vi "Ej_13_DAQ_Escritura_Digital.vi"() -> ()   [LabVIEW 2021]
panel:
  in  "lower limit":dbl
  in  "upper limit":dbl
  out "Temperatura":dbl
  in  "stop":bool
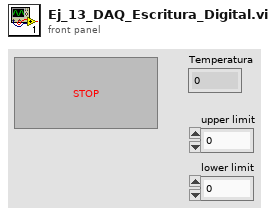
[diagram p1: front panel]
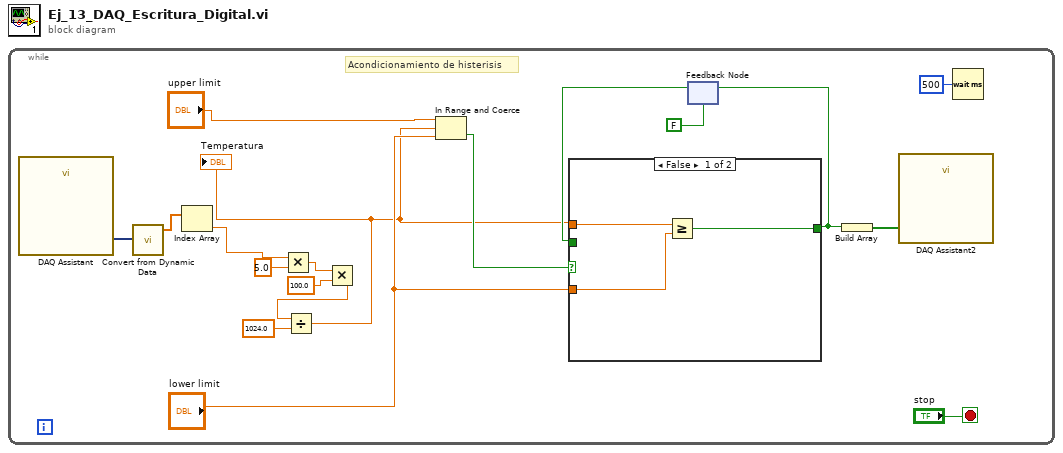
[diagram p0: block diagram]
diagram:
  n1 = while {
    stop <- "stop" stop-if-true
    # "Acondicionamiento de histerisis"
    n2 = call "DAQ Assistant"() -> ("data"=w13:dynamicdata)  [unwired: 17 in, 2 out]
    n3 = call "Convert from Dynamic Data"("Dynamic Data Type"=w13) -> ("Array"=w12:dbl[])  [unwired: 3 in]
    n4 = Index Array(array=w12) -> (element=w2:dbl)  [unwired: 1 in]
    n5 = Multiply(x=w2, y=5.0) -> (x*y=w6:dbl)
    n6 = Multiply(x=w6, y=100.0) -> (x*y=w4:dbl)
    n7 = Divide(x=w4, y=1024.0) -> (x/y=w1:dbl)
    "Temperatura" <- w1
    n8 = In Range and Coerce(upper limit="upper limit", x=w1, lower limit="lower limit") -> (In Range?=w16:bool)  [unwired: 1 out]
    n9 = feedback #1(FALSE) -> (w15:bool)
    n10 = case shown="False" w16 {
      tunnel: w1 -> [w21 _]
      tunnel: "lower limit" -> [w20 _]
      tunnel: [w19 w22] -> w11
      tunnel: w15 -> [_ w22]
      frame False {
        n11 = Greater Or Equal?(x=w21, y=w20) -> (x >= y?=w19:bool)
      }
      frame True {
      }
    }
    n12 = feedback-in #1(w11) -> ()
    n13 = Build Array(w11) -> (w10:bool[])
    n14 = call "DAQ Assistant2"("data"=w10) -> ()  [unwired: 17 in, 2 out]
    n15 = Wait (ms)(milliseconds to wait=u32 500) -> ()  [unwired: 1 out]
  }
